vi "CtlToJson.vi"(6 "JSON Origin Path":path, 7 "App Ref":refnum<vi>, 8 "error (in)":errorcluster, 9 "VI Origin Path":path, 10 "Destination Directory":path, 11 "VI Path":path) -> (0 "error out":errorcluster, 2 "JSON File Path":path, 3 "JSON":string)   [LabVIEW 2017]
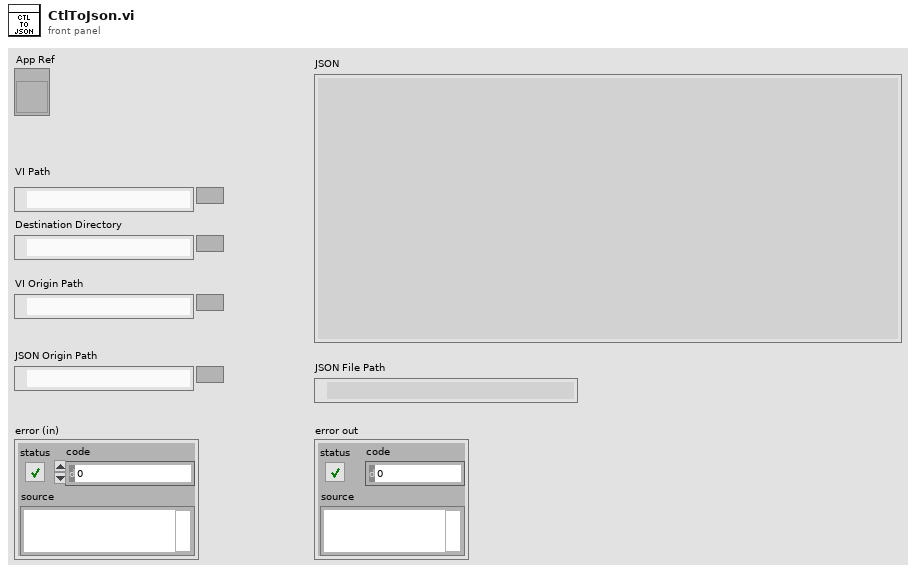
[diagram p1: front panel]
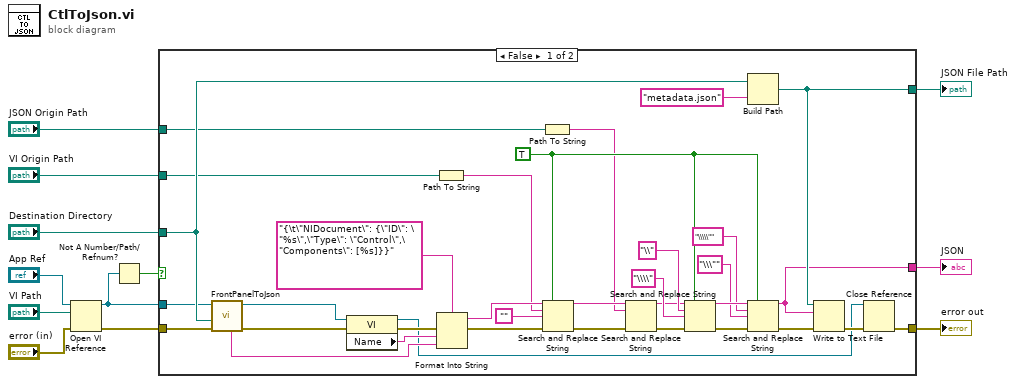
[diagram p0: block diagram]
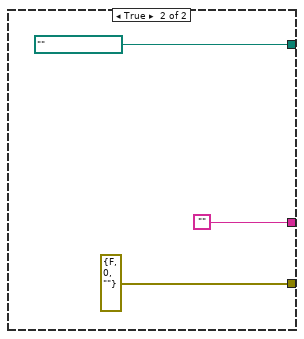
[diagram p2: hidden frame]
diagram:
  n1 = Open VI Reference(application reference (local)="App Ref", vi path="VI Path", error in (no error)="error (in)") -> (vi reference=w7:refnum<vi>, error out=w9:errorcluster)  [unwired: 3 in]
  n2 = Not A Number/Path/Refnum?(number/path/refnum=w7) -> (NaN/Path/Refnum?=w5:bool)
  n3 = case shown="False" w5 {
    tunnel: [w46 path ""] -> w12
    tunnel: [w23 errorcluster {"status"=FALSE, "code"=0, "source"=""} ("error out")] -> w11
    tunnel: w9 -> [w43 _]
    tunnel: "Destination Directory" -> [w45 _]
    tunnel: w7 -> [w44 _]
    tunnel: "VI Origin Path" -> [w15 _]
    tunnel: "JSON Origin Path" -> [w14 _]
    tunnel: [w13 ""] -> w2
    frame False {
      w29 = TRUE ("replace all? (F)")
      n4 = call "FrontPanelToJson.vi"("error in"=w43, "JSON Path"=w45, "VI in"=w44) -> ("error out"=w34:errorcluster, "VI out"=w28:refnum<vi>, "JSON"=w35:string)  [unwired: 5 in]
      n5 = property class="VI"(reference=w28, error in=w34) -> (reference out=w22:refnum<vi>, error out=w38:errorcluster, "Name"=w27:string)
      n6 = Path To String(path=w15) -> (string=w21:string)
      n7 = Format Into String(format string="{\t\"NIDocument\": {\"ID\": \"%s\",\"Type\": \"Control\",\"Components\": [%s]}}", error in=w38, w27, w35) -> (resulting string=w40:string, error out=w37:errorcluster)  [unwired: 1 in]
      n8 = Path To String(path=w14) -> (string=w17:string)
      n9 = Search and Replace String(replace all?=w29, input string=w40, search string=w21, replace string="", error in=w37) -> (result string=w18:string, error out=w20:errorcluster)  [unwired: 3 in, 2 out]
      n10 = Search and Replace String(input string=w18, search string=w17, error in=w20) -> (result string=w16:string, error out=w19:errorcluster)  [unwired: 5 in, 2 out]
      n11 = Search and Replace String(replace all?=w29, input string=w16, search string="\\", replace string="\\\\" ("replace string (\"\")"), error in=w19) -> (result string=w33:string, error out=w30:errorcluster)  [unwired: 3 in, 2 out]
      n12 = Build Path(base path=w45, name or relative path="metadata.json") -> (appended path=w46:path)
      n13 = Search and Replace String(replace all?=w29, input string=w33, search string="\\\\\"", replace string="\\\"" ("replace string (\"\")"), error in=w30) -> (result string=w13:string, error out=w26:errorcluster)  [unwired: 3 in, 2 out]
      n14 = Write to Text File(file (use dialog)=w46, text=w13, error in=w26) -> (error out=w24:errorcluster)  [unwired: 1 in, 2 out]
      n15 = Close Reference(reference=w22, error in (no error)=w24) -> (error out=w23:errorcluster)
    }
    frame True {
    }
  }
  "JSON File Path" <- w12
  "error out" <- w11
  "JSON" <- w2
